vi "SSL Detection Frame Robots Kalman Estimator.vi"(0 "Lado":enum16{"Esquerdo", "Direito"}(ring) caption="Enum", 5 "Time Stamp":timestamp, 6 "our_robots":bool=TRUE, 7 "Life Time":dbl=1.0, 8 "ignora esquerda?":bool=TRUE, 9 "ignora lado":bool, 10 "our_robots":T1[](array[typedef]), 11 "Robots":T6[](array[typedef]) {"height" format="%+4.3f"; "pixel_y" format="%+4.3f"; "pixel_x" format="%+4.3f"; "orientation" format="%+4.3f"; "y" format="%+4.3f"; "confidence" format="%4.3f"; "x" format="%+4.3f"}) -> (3 "Robots Out":T6[](array[typedef]) {"height" format="%+4.3f"; "pixel_y" format="%+4.3f"; "pixel_x" format="%+4.3f"; "orientation" format="%+4.3f"; "y" format="%+4.3f"; "confidence" format="%4.3f"; "x" format="%+4.3f"})   [LabVIEW 2017]
uses:
  SSL Detection Robot.ctl
  <vilib>/Analysis/Matrix/Datatypes/RealMatrix.ctl
  Core/AI Robot.ctl
  Intel/Functions Enum.ctl
  Intel/AttackerStates.ctl
  Path Planning/RRT/PathDests.ctl
  Path Planning/RRT/PathDest.ctl
  <vilib>/Analysis/coordinate.llb/Wrap Angle (scalar).vi
  <vilib>/Analysis/_algsub.llb/Real Vector Norm.vi
  <vilib>/Analysis/Matrix/Numeric/Conversions/Array To Matrix - RA.vi
  <vilib>/Analysis/Matrix/Numeric/Subtract/Subtract - RM,RM.vi
  <vilib>/Analysis/NI_AALPro.lvlib
  <vilib>/Analysis/Matrix/NI_Matrix.lvlib
  <vilib>/Analysis/NI_AAL_Angle.lvlib
panel:
  in  "Robots Out 2":T8(array[cluster]) {"Detection Robot"."height" format="%+4.3f"; "Detection Robot"."pixel_y" format="%+4.3f"; "Detection Robot"."pixel_x" format="%+4.3f"; "Detection Robot"."orientation" format="%+4.3f"; "Detection Robot"."y" format="%+4.3f"; "Detection Robot"."confidence" format="%4.3f"; "Detection Robot"."x" format="%+4.3f"}
  out "A-B":dbl[][](array[numeric])
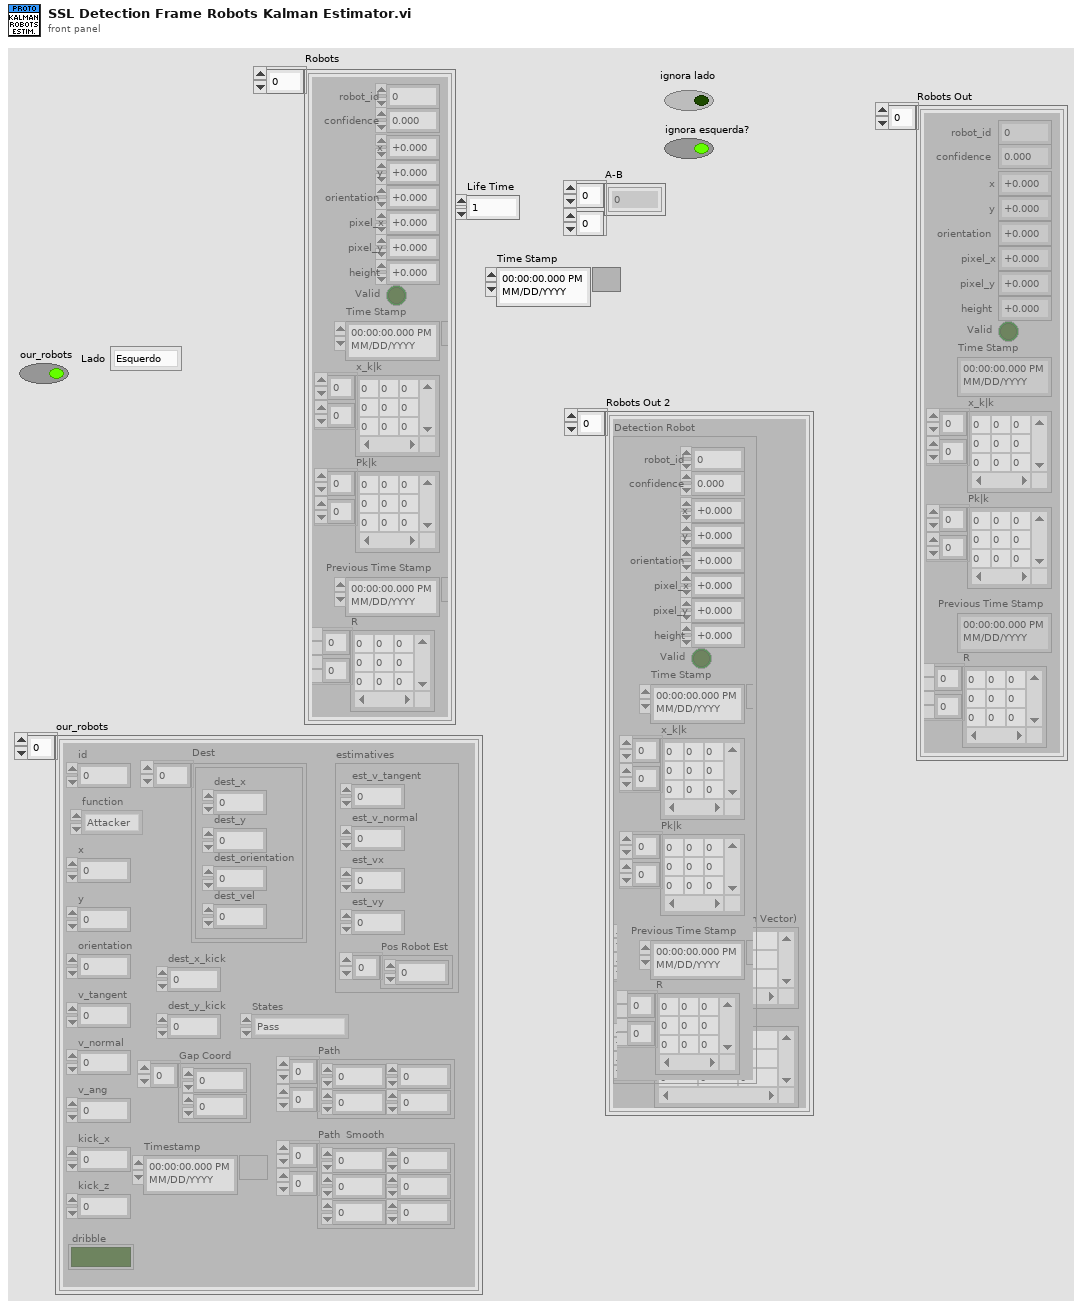
[diagram p1: front panel]
types:
  T1 = typedef "AI Robot.ctl" = cluster{"id":u32, "function":T2, "x":dbl, "y":dbl, "orientation":dbl, "v_tangent":dbl, "v_normal":dbl, "v_ang":dbl, "kick_x":dbl, "kick_z":dbl, "dribble":bool, "Timestamp":timestamp, "estimatives":cluster{"est_v_tangent":dbl, "est_v_normal":dbl, "est_vx":dbl, "est_vy":dbl, "Pos Robot Est":dbl[]}, "dest_x_kick":dbl, "dest_y_kick":dbl, "Gap Coord":dbl[], "States":T3, "Path ":dbl[][], "Path  Smooth":dbl[][], "Dest":T4}
  T2 = typedef "Functions Enum.ctl" = enum16{"Attacker", "Goalie", "Defender", "Striker", "Goto 0", "Dummy", "Kicker", "ZigZag"}
  T3 = typedef "AttackerStates.ctl" = enum16{"Pass", "GoToTangent", "BallGetting", "GoToKick", ""}
  T4 = typedef "PathDests.ctl" = T5[]
  T5 = typedef "PathDest.ctl" = cluster{"dest_x":dbl, "dest_y":dbl, "dest_orientation":dbl, "dest_vel":dbl}
  T6 = typedef "SSL Detection Robot.ctl" = cluster{"x":sgl, "robot_id":u32, "confidence":sgl, "y":sgl, "orientation":sgl, "pixel_x":sgl, "pixel_y":sgl, "height":sgl, "Valid":bool, "Time Stamp":timestamp, "x_k|k":T7, "Pk|k":T7, "Previous Time Stamp":timestamp, "R":T7}
  T7 = typedef "NI_Matrix.lvlib/RealMatrix.ctl" = dbl[][]
  T8 = cluster{"Detection Robot":T6, "Real Matrix (Column Vector)":T7, "Pk|k":T7}[]
  T9 = cluster{"Detection Robot":T6, "Real Matrix (Column Vector)":T7, "Pk|k":T7}
  T10 = cluster{"Detection Robot out":T6, "x_k|k":T7, "Pk|k":T7}
  T11 = typedef "SSL Detection Robot.ctl" = cluster{"x":sgl, "robot_id":u32, "confidence":sgl, "y":sgl, "orientation":sgl, "pixel_x":sgl, "pixel_y":sgl, "height":sgl, "Valid":bool, "Time Stamp":timestamp, "x_k|k":T7, "Pk|k":T7}
  T12 = cluster{"Detection Robot":T11, "Real Matrix (Column Vector)":T7, dbl[][]}
  T13 = cluster{"Detection Robot out":T6, "x_k|k":T7, "Pk|k":T7}[]
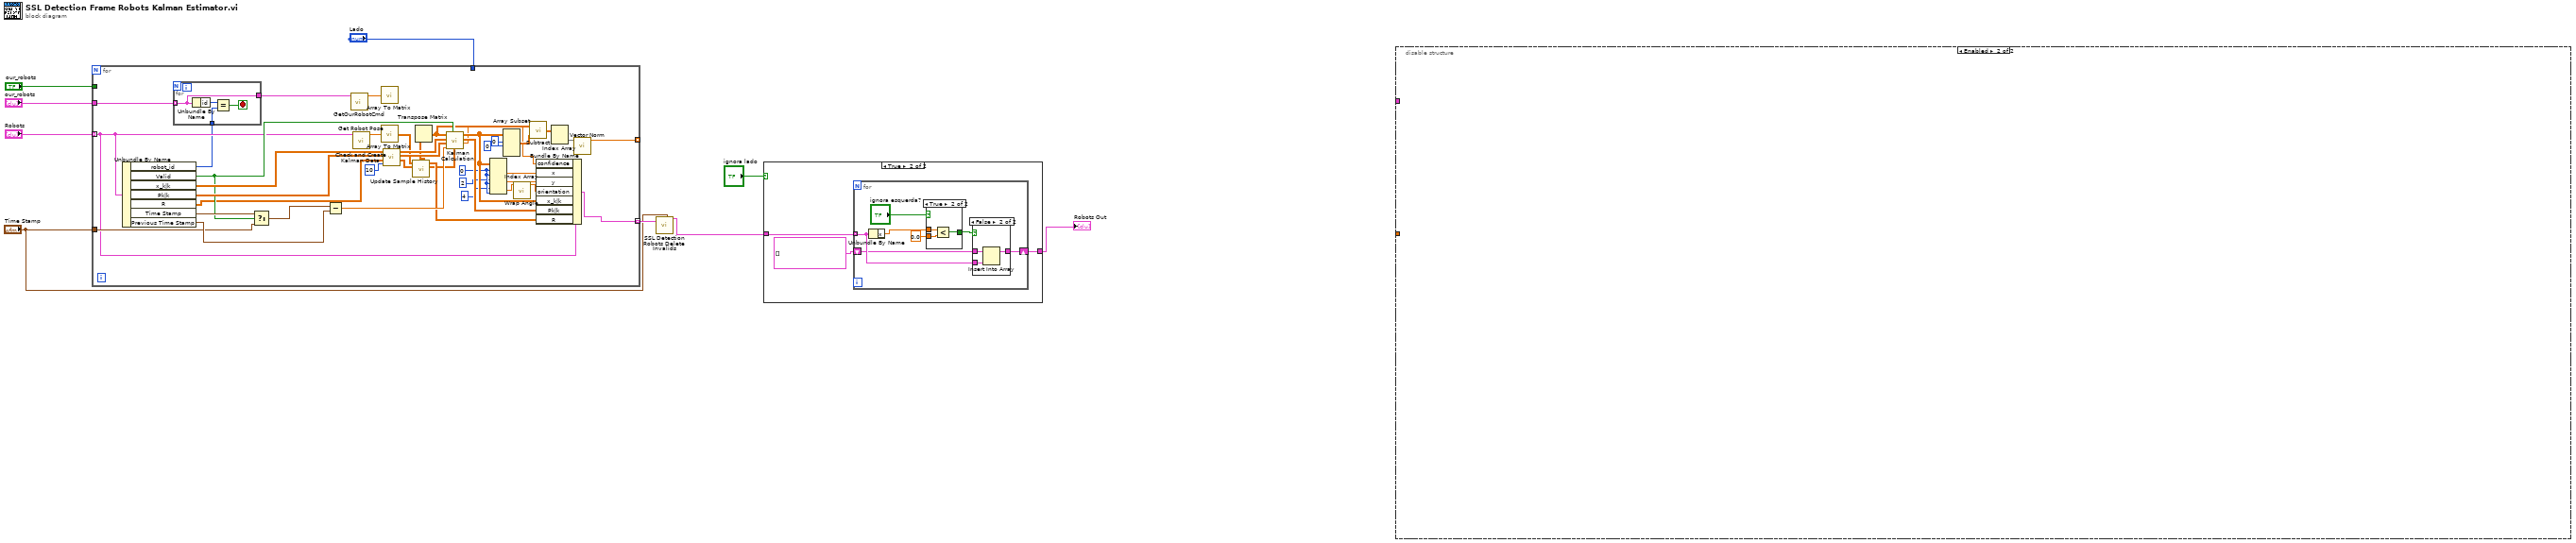
[diagram p0: block diagram]
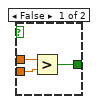
[diagram p3: hidden frame]
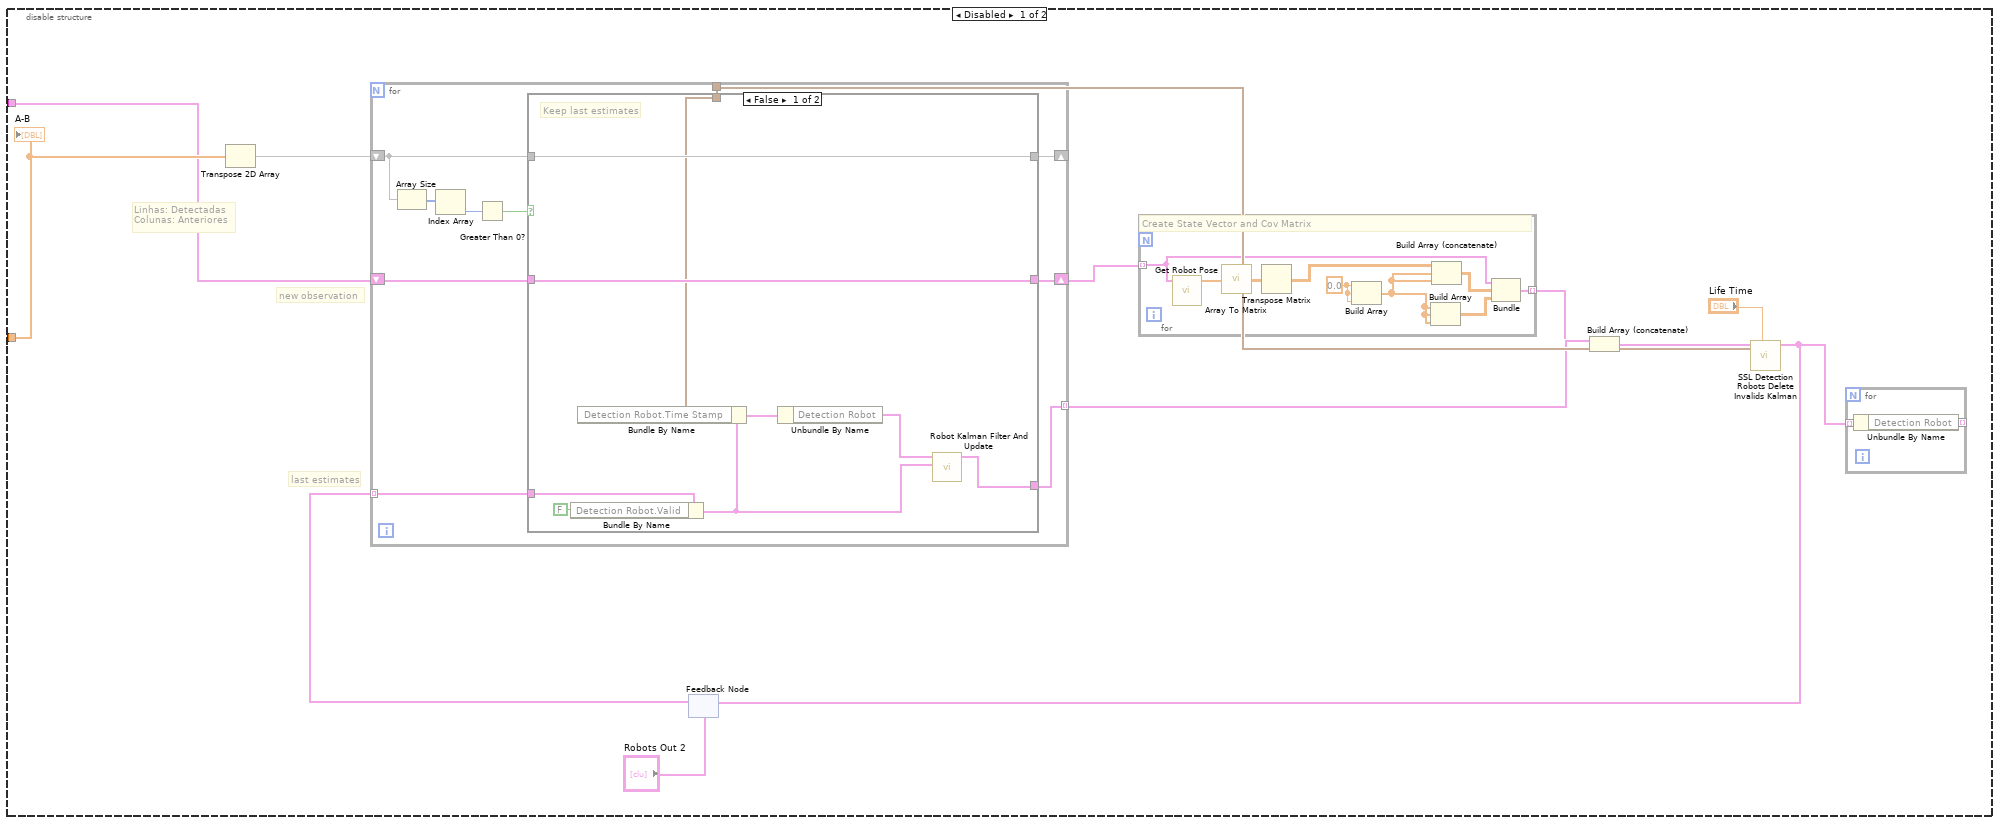
[diagram p5: hidden frame]
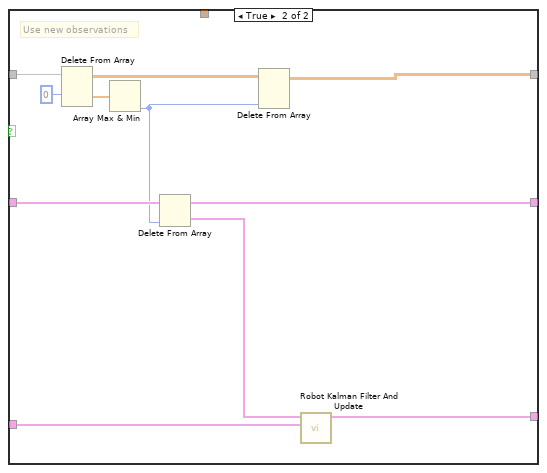
[diagram p6: hidden frame]
diagram:
  n1 = for {
    tunnel: "Robots" -> [w32] mode=indexing
    tunnel: [w50] -> _ mode=indexing
    tunnel: [w14] -> w8 mode=indexing
    tunnel: "Time Stamp" -> [w35]
    tunnel: "our_robots" -> [w13]
    tunnel: "our_robots" -> [_]
    tunnel: "Lado" -> [_]
    w28 = 0 ("index (row)")
    n2 = Unbundle By Name(w32) -> ("robot_id"=w12:u32, "Valid"=w33:bool, "x_k|k"=w42:T7, "Pk|k"=w40:T7, "R"=w25:T7, "Time Stamp"=w36:timestamp, "Previous Time Stamp"=w38:timestamp)
    n3 = for {
      tunnel: w13 -> [w51] mode=indexing
      tunnel: w12 -> [w52]
      tunnel: [w51] -> w11
      stop <- w54 stop-if-true
      n4 = Unbundle By Name(w51) -> ("id"=w53:u32)
      n5 = Equal?(x=w53, y=w52) -> (x = y?=w54:bool)
    }
    n6 = Select(t=w36, s=w33, f=w35) -> (s? t:f=w34:timestamp)
    n7 = Subtract(x=w34, y=w38) -> (x-y=w37:dbl)
    n8 = call "GetOurRobotCmd.vi"("Robot"=w11) -> ("Vel"=w10:dbl[])  [unwired: 10 in]
    n9 = call "Get Robot Pose.vi"("Detection Robot"=w32) -> ("Pose"=w44:sgl[])  [unwired: 10 in]
    n10 = call-poly <vilib>:"Array To Matrix.vi"("Real 1D Array"=w10) -> ()  [unwired: 1 out]
    n11 = call-poly <vilib>:"Array To Matrix.vi"("Real 1D Array"=w44) -> ("Real Matrix (Column Vector)"=w21:T7)
    n12 = call "Check and Create Kalman Data.vi"("Variance Memory"=10, "R"=w25, "Pk"=w40, "x_k"=w42) -> ("R out"=w24:T7, "Pk out"=w39:T7, "x_k out"=w41:T7)  [unwired: 5 in]
    n13 = call "Update Sample History.vi"("R in"=w24, "Sample"=w21) -> ("covariance matrix V"=w19:T7, "R out"=w20:T7, "Sample Unwrapped"=w18:T7)  [unwired: 7 in]
    n14 = Transpose Matrix(1:w18) -> (0:w22:T7)
    n15 = call "Kalman Calculation.vi"("R"=w19, "Use Observation"=w33, "intervalo"=w37, "Pk-1|k-1"=w39, "x_k-1|k-1"=w41, "z_k"=w22) -> ("Conf"=w15:dbl, "Pk|k"=w43:T7, "x_k|k"=w31:T7)  [unwired: 3 in]
    n16 = Index Array(array=w31, index (row) #1=w28, index (col) #1=w28, index (row) #2=2 ("disabled index (col)"), index (col) #2=w28, index (row) #3=4 ("disabled index (col)"), index (col) #3=w28) -> (element #1=w30:dbl, element #2=w29:dbl, element #3=w17:dbl)
    n17 = Array Subset(array=w31, index (row)=0 ("row 1"), length (row)=0 ("row N")) -> (w49:T7)  [unwired: 2 in]
    n18 = call-poly <vilib>:"Wrap Angle.vi"("angle in"=w17) -> ("angle out"=w16:dbl)  [unwired: 9 in, 1 out]
    n19 = call-poly <vilib>:"Subtract.vi"("Real Matrix B"=w49, "Real Matrix A"=w22) -> ("A - B"=w46:T7)
    n20 = Bundle By Name(cluster=w32, "confidence"=w15, "x"=w30, "y"=w29, "orientation"=w16, "x_k|k"=w31, "Pk|k"=w43, "R"=w20) -> (w14:T6)
    n21 = Index Array(array=w46) -> (element=w45:dbl[])  [unwired: 2 in]
    n22 = call-poly <vilib>:"Vector Norm.vi"("Input Vector"=w45) -> ("norm"=w50:dbl)  [unwired: 9 in, 1 out]
  }
  n23 = call "SSL Detection Robots Delete Invalids.vi"("Now"="Time Stamp", "Robots In"=w8) -> ("Robots Out"=w5:T6[])  [unwired: 9 in]
  n24 = case shown="True" "ignora lado" {
    tunnel: w5 -> [w55 w58]
    tunnel: [w55 w56] -> w4
    frame False {
    }
    frame True {
      n25 = for {
        tunnel: w58 -> [w65] mode=indexing
        shift-right: [w59] -> w56
        shift-left: T6[] [] ("Robots Out") -> [w60]
        n26 = Unbundle By Name(w65) -> ("x"=w64:sgl)
        n27 = case shown="True" "ignora esquerda?" {
          tunnel: w64 -> [w68 w71]
          tunnel: sgl 0.0 ("y") -> [w67 w70]
          tunnel: [w66 w69] -> w62
          frame False {
            n28 = Greater?(x=w68, y=w67) -> (0:w66:bool)
          }
          frame True {
            n29 = Less?(x=w71, y=w70) -> (x < y?=w69:bool)
          }
        }
        n30 = case shown="False" w62 {
          tunnel: w65 -> [_ w74]
          tunnel: [w72 w75] -> w59
          tunnel: w60 -> [w72 w73]
          frame True {
          }
          frame False {
            n31 = Insert Into Array(array=w73, new element=w74) -> (w75:T6[])  [unwired: 1 in]
          }
        }
      }
    }
  }
  "Robots Out" <- w4
  n32 = disable-structure shown="Enabled" {
    disable-tunnel: _ -> [w84 _]
    disable-tunnel: _ -> [w83 _]
    frame Disabled {
      # "Linhas: Detectadas\nColunas: Anteriores"
      # "last estimates"
      # "new observation"
      n33 = Transpose 2D Array(2D array=w84) -> (transposed array=w85:dbl[][])
      n34 = feedback #1("Robots Out 2") -> (w77:T8)
      n35 = for {
        shift-right: [w107] -> _
        shift-left: w85 -> [w103]
        shift-right: [w106] -> w82
        shift-left: w83 -> [w108]
        tunnel: [w105] -> w81 mode=indexing
        tunnel: w77 -> [w104] mode=indexing
        tunnel: [w99] -> w86
        n36 = Array Size(array=w103) -> (size(s)=w101:i32[])
        n37 = Index Array(array=w101) -> (element=w100:i32)  [unwired: 1 in]
        n38 = Greater Than 0?(x=w100) -> (x > 0?=w102:bool)
        n39 = case shown="False" w102 {
          tunnel: w103 -> [w117 w128]
          tunnel: w108 -> [w116 w125]
          tunnel: [w117 w123] -> w107
          tunnel: [w116 w121] -> w106
          tunnel: [w112 w120] -> w105
          tunnel: w104 -> [w111 w118]
          tunnel: w99 -> [w114 _]
          frame False {
            # "Keep last estimates"
            n40 = Bundle By Name(cluster=w111, "Detection Robot.Valid"=FALSE ("Detection Ball.Valid")) -> (w109:T9)
            n41 = Bundle By Name(cluster=w109, "Detection Robot.Time Stamp"=w114) -> (w113:T9)
            n42 = Unbundle By Name(w113) -> ("Detection Robot"=w110:T6)
            n43 = call "Robot Kalman Filter And Update.vi"("Cluster in"=w109, "Detection Robot"=w110) -> ("Cluster out"=w112:T10)  [unwired: 9 in]
          }
          frame True {
            # "Use new observations"
            n44 = Delete From Array(array=w128, index (row)=0) -> (deleted portion=w126:dbl[], array with subset deleted=w124:dbl[][])  [unwired: 2 in]
            n45 = Array Max & Min(array=w126) -> (min index (indices)=w122:i32)  [unwired: 3 out]
            n46 = Delete From Array(array=w125, index=w122) -> (deleted portion=w119:T11, array with subset deleted=w121:T11[])  [unwired: 1 in]
            n47 = Delete From Array(array=w124, index (col)=w122) -> (array with subset deleted=w123:dbl[][])  [unwired: 2 in, 1 out]
            n48 = call "Robot Kalman Filter And Update.vi"("Cluster in"=w118, "Detection Robot"=w119) -> ("Cluster out"=w120:T10)  [unwired: 9 in]
          }
        }
      }
      n49 = for {
        tunnel: w82 -> [w91] mode=indexing
        tunnel: [w94] -> w80 mode=indexing
        w98 = 0.0 ("element")
        # "Create State Vector and Cov Matrix"
        n50 = call "Get Robot Pose.vi"("Detection Robot"=w91) -> ("Pose"=w93:sgl[])  [unwired: 10 in]
        n51 = call-poly <vilib>:"Array To Matrix.vi"("Real 1D Array"=w93) -> ("Real Matrix (Column Vector)"=w92:T7)
        n52 = Transpose Matrix(1:w92) -> (0:w90:T7)
        n53 = Build Array(w98, w98, w98) -> (w97:dbl[])
        n54 = Build Array(w97, w97, w97) -> (w96:dbl[][])
        n55 = Build Array (concatenate)(w90, w97, w97) -> (w95:T7)
        n56 = Bundle("Detection Robot"=w91, "Real Matrix (Column Vector)"=w95, w96) -> (w94:T12)  [unwired: 1 in]
      }
      n57 = Build Array (concatenate)(w81, w80) -> (w76:T13)
      n58 = call "SSL Detection Robots Delete Invalids Kalman.vi"("Now"=w86, "Life Time"="Life Time", "Robots In"=w76) -> ("Robots Out"=w79:T8)  [unwired: 8 in]
      n59 = feedback-in #1(w79) -> ()
      n60 = for {
        tunnel: w79 -> [w89] mode=indexing
        tunnel: [w88] -> _ mode=indexing
        n61 = Unbundle By Name(w89) -> ("Detection Robot"=w88:T6)
      }
      "A-B" <- w84
    }
    frame Enabled {
    }
  }
